vi "CPU Usage of Loop.vi"() -> ()   [LabVIEW 2020]
panel:
  in  "stop":bool
  out "y":dbl
  in  "Y-Intercept (b)":dbl
  in  "x":dbl
  in  "Slope (m)":dbl
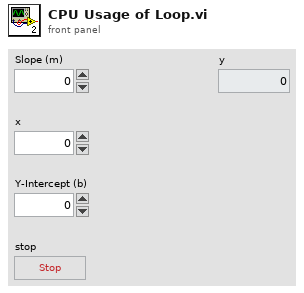
[diagram p1: front panel]
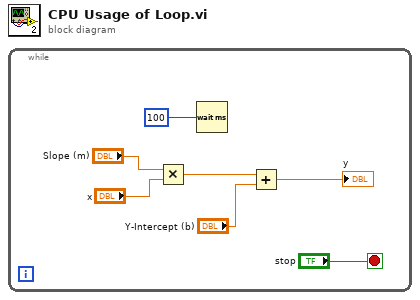
[diagram p0: block diagram]
diagram:
  n1 = while {
    stop <- "stop" stop-if-true
    n2 = Multiply(x="Slope (m)", y="x") -> (x*y=w5:dbl)
    n3 = Wait (ms)(milliseconds to wait=u32 100) -> ()  [unwired: 1 out]
    n4 = Add(x=w5, y="Y-Intercept (b)") -> (x+y=→"y":dbl)
  }
